vi "STM32 Com.vi"() -> ()   [LabVIEW 2025]
doc: "This example performs writes and reads on a serial port, as directed by the user. You can press the Write and Read buttons, and change the Read Count, while the example is running.\n\nThe parameters set for the serial port must match the parameters of the connected instrument or device. In this example, the Read Count parameter specifies the number of bytes that the serial port reads. If there were more bytes at the port than the specified number, those bytes would not be read. If there were less bytes at the port than the specified number, you would receive a timeout error.\n\nThis example expands upon the flow control options for XON and XOFF, allowing the user to choose those control characters. Also, the user can enable or disable a termination character. Some devices require a termination character in order to identify the end of command strings. Some devices send a termination character to signify the end of data to be read. This example shows how you can end the Read operation once a termination character is detected in the buffer and/or append a termination character at the end of the Write data."
uses:
  support/Serial - Settings.ctl
  <vilib>/Instr/_visa.llb/VISA Configure Serial Port (Instr).vi
panel:
  out "Temp":dbl
  out "Desired Temp":dbl
  out "PWM":u32
  out "Gas":u32
  out "Light":u32
  in  "Termination Character":u8=10 format="%.0x"
  in  "End Write on Termination Character?":bool=TRUE
  in  "Stop":bool
  in  "Command":string="*IDN?"
  in  "Read Count":u32=1000
  out "Response":string
  in  "Write":bool
  in  "Read":bool
  in  "Serial Settings":T1={"baud rate"=9600, "data bits"=8, "parity"=enum."None", "stop bits"=10, "flow control"=0} {"flow control" items=["None"=0, "XON/XOFF"=1, "RTS/CTS"=2, "DTR/DSR"=4]; "stop bits" items=["1.0"=10, "1.5"=15, "2.0"=20]; "data bits" min=5 max=8 step=1; "baud rate" items=["75"=75, "110"=110, "134"=134, "150"=150, "300"=300, "600"=600, "1200"=1200, "1800"=1800, "2400"=2400, "4800"=4800, "7200"=7200, "9600"=9600, "14400"=14400, "19200"=19200, "28800"=28800, "38400"=38400, "56000"=56000, "57600"=57600, "115200"=115200, "128000"=128000, "230400"=230400]}
  in  "End Read on Termination Character?":bool=TRUE
  # "0xA is equivalent to a '\\n' character, which is a line feed."
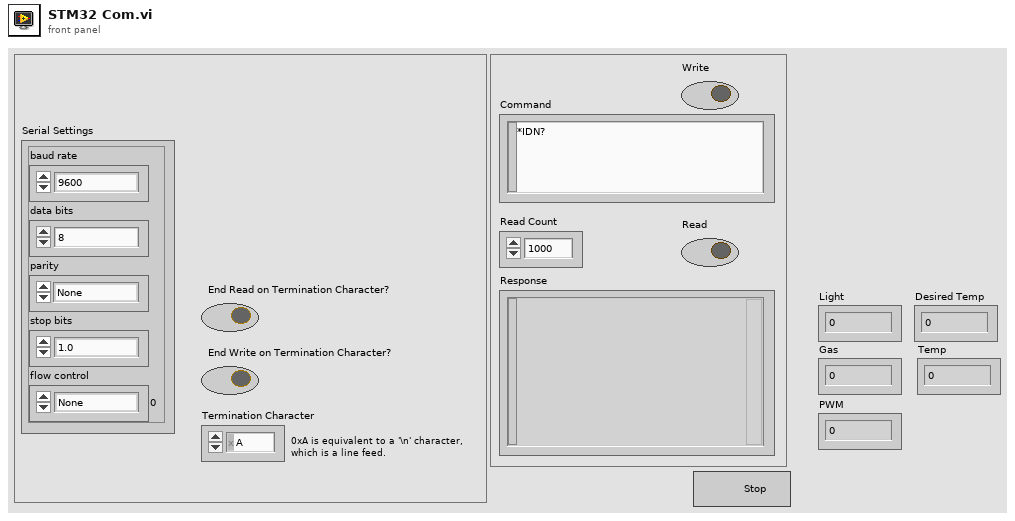
[diagram p1: front panel]
types:
  T1 = typedef "Serial - Settings.ctl" = cluster{"baud rate":u32, "data bits":u16, "parity":enum16{"None", "Odd", "Even", "Mark", "Space"}, "stop bits":u16, "flow control":u16}
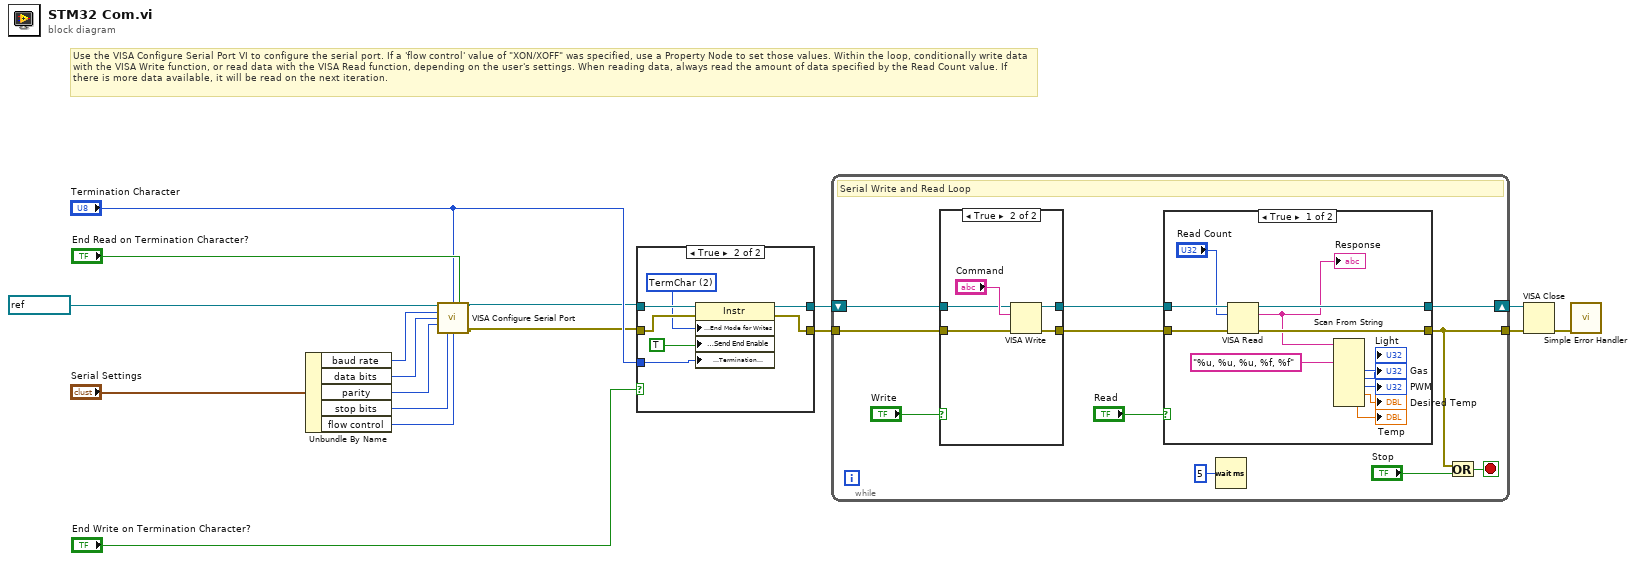
[diagram p0: block diagram]
diagram:
  # "Use the VISA Configure Serial Port VI to configure the serial port. If a 'flow control' value of \"XON/XOFF\" was specified, use a Property Node to set those values. Within the loop, conditionally write data with the VISA Write function, or read data with the VISA Read function, depending on the user's settings. When reading data, always read the amount of data specified by the Read Count value. If there is more data available, it will be read on the next iteration."
  n1 = Unbundle By Name("Serial Settings") -> ("baud rate"=w13:u32, "data bits"=w14:u16, "parity"=w15:enum16{"None", "Odd", "Even", "Mark", "Space"}, "stop bits"=w16:u16, "flow control"=w3:u16)
  n2 = call-poly "VISA Configure Serial Port"("VISA resource name"=refnum<visa-resource-name> "COM3", "termination char\n(0xA = '\\n' = LF)"="Termination Character", "Enable Termination\nChar (T)"="End Read on Termination Character?", "baud rate (9600)"=w13, "data bits (8)"=w14, "parity (0:none)"=w15, "stop bits (10: 1 bit)"=w16, "flow control (0:none)"=w3) -> ("VISA resource name out"=w2:refnum<visa-resource-name>, "error out"=w1:errorcluster)  [unwired: 2 in, 4 out]
  n3 = case shown="True" "End Write on Termination Character?" {
    tunnel: w2 -> [w18 w26]
    tunnel: w1 -> [w19 w25]
    tunnel: [w18 w24] -> w6
    tunnel: [w19 w23] -> w7
    tunnel: "Termination Character" -> [_ w21]
    frame False {
    }
    frame True {
      w22 = u16 2 items=["None", "LastBit", "TermChar", "Break"] ("Serial Settings:Serial End Mode for Writes")
      n4 = property class="Instr"(reference=w26, error in=w25, "Serial Settings:End Mode for Writes"=w22, "Message Based Settings:Send End Enable"=TRUE, "Message Based Settings:Termination Character"=w21) -> (reference out=w24:refnum<visa-resource-name>, error out=w23:errorcluster)
    }
  }
  n5 = while {
    shift-right: [w37] -> w8
    shift-left: w6 -> [w36]
    tunnel: w7 -> [w35]
    tunnel: [w29] -> w9
    stop <- w30 stop-if-true
    # "Serial Write and Read Loop"
    n6 = case shown="True" "Write" {
      tunnel: w36 -> [w39 w43]
      tunnel: w35 -> [w38 w42]
      tunnel: [w39 w41] -> w34
      tunnel: [w38 w40] -> w33
      frame False {
      }
      frame True {
        n7 = VISA Write(VISA resource name=w43, write buffer="Command", error in (no error)=w42) -> (VISA resource name out=w41:refnum<visa-resource-name>, error out=w40:errorcluster)  [unwired: 1 out]
      }
    }
    n8 = case shown="True" "Read" {
      tunnel: [w54 w58] -> w37
      tunnel: w34 -> [w56 w58]
      tunnel: [w52 w57] -> w29
      tunnel: w33 -> [w55 w57]
      frame True {
        n9 = VISA Read(VISA resource name=w56, byte count="Read Count", error in (no error)=w55) -> (VISA resource name out=w54:refnum<visa-resource-name>, read buffer=w51:string, error out=w52:errorcluster)  [unwired: 1 out]
        "Response" <- w51
        n10 = Scan From String(format string="%u, %u, %u, %f, %f", input string=w51) -> (output 1=→"Light":u32, output 2=→"Gas":u32, output 3=→"PWM":u32, output 4=→"Desired Temp":dbl, output 5=→"Temp":dbl)  [unwired: 7 in, 3 out]
      }
      frame False {
      }
    }
    n11 = Wait (ms)(milliseconds to wait=u32 5) -> ()  [unwired: 1 out]
    n12 = Or(x=w29, y="Stop") -> (x .or. y?=w30:bool)
  }
  n13 = VISA Close(VISA resource name=w8, error in (no error)=w9) -> (error out=w10:errorcluster)
  n14 = call <vilib>:"Simple Error Handler.vi"("error in (no error)"=w10) -> ()  [unwired: 1 in, 8 out]
